vi "GetText.vi"(8 "error in":errorcluster, 11 "GPIC ScaleAndLimit editor node in":refnum<class "GPIC ScaleAndLimit editor node.lvclass">) -> (0 "error out":errorcluster, 1 "additional text":string, 2 "text":string, 3 "GPIC ScaleAndLimit editor node out":refnum<class "GPIC ScaleAndLimit editor node.lvclass">, 4 "glyph":string)   [LabVIEW 2015, in "GPIC ScaleAndLimit editor node.lvclass"]
uses:
  GPIC ScaleAndLimit editor node.lvclass
  <vilib>/NI/DCAF/Tag Editor Core/control module/editor node/control module editor.lvclass
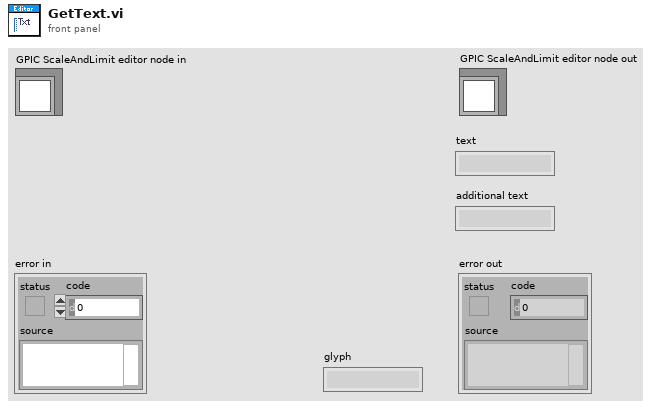
[diagram p1: front panel]
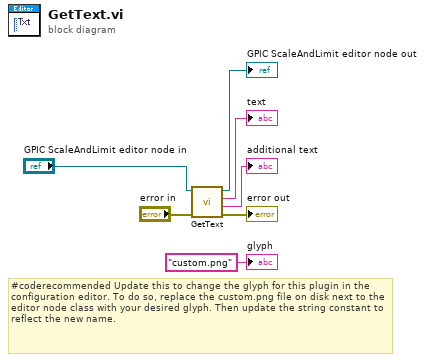
[diagram p0: block diagram]
diagram:
  # "#coderecommended Update this to change the glyph for this plugin in the configuration editor. To do so, replace the custom.png file on disk next to the editor node class with your desired glyph. Then update the string constant to reflect the new name."
  n1 = call-parent "GetText.vi"("error in"="error in", "Module Editor Node in"="GPIC ScaleAndLimit editor node in") -> ("error out"=→"error out":errorcluster, "additional text"=→"additional text":string, "text"=→"text":string, "Module Editor Node out"=→"GPIC ScaleAndLimit editor node out":refnum<class "GPIC ScaleAndLimit editor node.lvclass">)  [unwired: 5 in, 1 out]
  "glyph" <- "custom.png" ("glyph")
